vi "allowedvis.vi"() -> (1 "AllowedVis":string[](array[string]), 2 "App.ExportedVIs":string[](array[string]))   [LabVIEW 2010]
panel:
  out "size(s) 2":i32
  out "size(s)":i32
  # "Все разрешенные вишки с контролами"
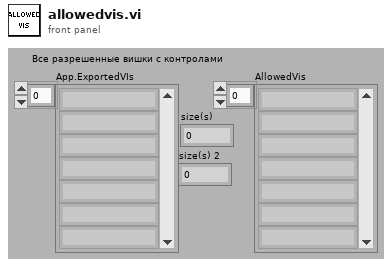
[diagram p1: front panel]
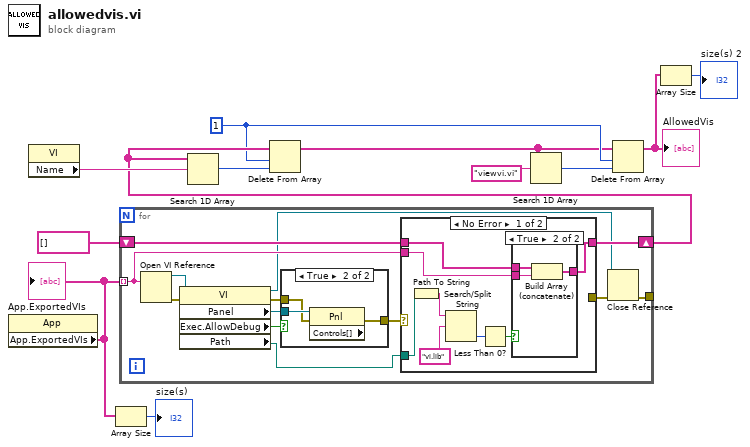
[diagram p0: block diagram]
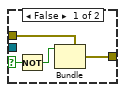
[diagram p2: hidden frame]
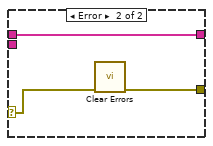
[diagram p4: hidden frame]
diagram:
  w7 = 1 ("length")
  n1 = property class="App"() -> ("App.ExportedVIs"=w4:string[])  [unwired: 2 in, 2 out]
  "App.ExportedVIs" <- w4
  n2 = property class="VI"() -> ("Name"=w9:string)  [unwired: 2 in, 2 out]
  n3 = Array Size(array=w4) -> (size(s)=→"size(s)":i32)
  n4 = for {
    tunnel: w4 -> [w16] mode=indexing
    shift-right: [w22] -> w8
    shift-left: string[] [] -> [w21]
    tunnel: [w13] -> _
    n5 = Open VI Reference(vi path=w16) -> (vi reference=w24:refnum<vi>, error out=w25:errorcluster)  [unwired: 5 in]
    n6 = property class="VI"(reference=w24, error in=w25) -> (reference out=w14:refnum<vi>, error out=w18:errorcluster, "Panel"=w19:refnum<vi>, "Exec.AllowDebug"=w20:bool, "Path"=w17:path)
    n7 = case shown="True" w20 {
      selector: w20 -> [w29 _]
      tunnel: [w26 w32] -> w23
      tunnel: w19 -> [_ w31]
      tunnel: w18 -> [w27 w30]
      frame False {
        n8 = Not(x=w29) -> (.not. x?=w28:bool)
        n9 = Bundle(cluster=w27, "status"=w28) -> (w26:errorcluster)  [unwired: 2 in]
      }
      frame True {
        n10 = property class="Pnl" props=["Controls[]"](reference=w31, error in=w30) -> (error out=w32:errorcluster)  [unwired: 2 out]
      }
    }
    n11 = case shown="No Error" w23 {
      selector: w23 -> [_ w46]
      tunnel: [w34 w47] -> w22
      tunnel: w21 -> [w35 w47]
      tunnel: w17 -> [w40 _]
      tunnel: w16 -> [w33 _]
      tunnel: [_ w45] -> w15
      frame No Error {
        n12 = Path To String(path=w40) -> (string=w39:string)
        n13 = Search/Split String(string=w39, search string/char (-)="vi.lib") -> (offset of match=w37:i32)  [unwired: 1 in, 2 out]
        n14 = Less Than 0?(x=w37) -> (x < 0?=w36:bool)
        n15 = case shown="True" w36 {
          tunnel: w35 -> [w41 w44]
          tunnel: [w41 w43] -> w34
          tunnel: w33 -> [_ w42]
          frame False {
          }
          frame True {
            n16 = Build Array (concatenate)(w44, w42) -> (w43:string[])
          }
        }
      }
      frame Error {
        n17 = call <vilib>:"Clear Errors.vi"("error in (no error)"=w46) -> ("error out"=w45:errorcluster)  [unwired: 6 in]
      }
    }
    n18 = Close Reference(reference=w14, error in (no error)=w15) -> (error out=w13:errorcluster)
  }
  n19 = Search 1D Array(1D array=w8, element=w9) -> (index of element=w6:i32)  [unwired: 1 in]
  n20 = Delete From Array(array=w8, length=w7, index=w6) -> (array with subset deleted=w5:string[])  [unwired: 1 out]
  n21 = Search 1D Array(1D array=w5, element="viewvi.vi") -> (index of element=w11:i32)  [unwired: 1 in]
  n22 = Delete From Array(array=w5, length=w7, index=w11) -> (array with subset deleted=w2:string[])  [unwired: 1 out]
  "AllowedVis" <- w2
  n23 = Array Size(array=w2) -> (size(s)=→"size(s) 2":i32)
